vi "ALEX.vi"(1 "Frame Number\n(starts with 1)":i32, 2 "ALEX?":bool, 3 "Shutter Enable":bool[](array[boolean])) -> (0 "Shutter State":bool[](array[boolean]))   [LabVIEW 2023, in "NI DAQ.lvlib" / "NI DAQ.lvclass"]
uses:
  NI DAQ.lvclass
  NI DAQ.lvclass/NI DAQ.ctl
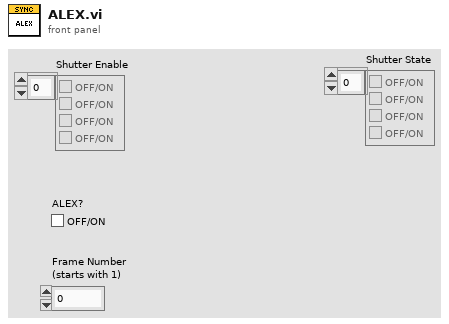
[diagram p1: front panel]
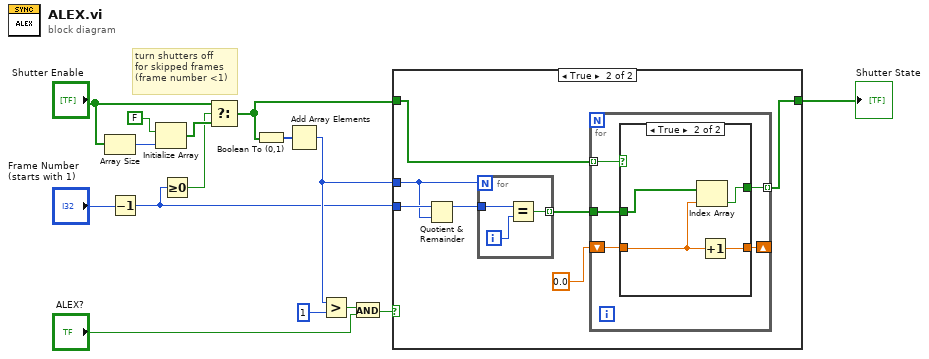
[diagram p0: block diagram]
diagram:
  # "turn shutters off\nfor skipped frames\n(frame number <1)"
  n1 = Array Size(array="Shutter Enable") -> (size(s)=w4:i32)
  n2 = Decrement(x="Frame Number\n(starts with 1)") -> (x-1=w2:i32)
  n3 = Initialize Array(FALSE, w4) -> (w6:bool[])
  n4 = Greater Or Equal To 0?(x=w2) -> (x >= 0?=w1:bool)
  n5 = Select(t="Shutter Enable", s=w1, f=w6) -> (s? t:f=w7:bool[])
  n6 = Boolean To (0,1)(Boolean=w7) -> (0, 1=w14:i16[])
  n7 = Add Array Elements(numeric array=w14) -> (sum=w11:i16)
  n8 = Greater?(x=w11, y=i16 1) -> (0:w12:bool)
  n9 = And(x=w12, y="ALEX?") -> (x .and. y?=w13:bool)
  n10 = case shown="True" w13 {
    tunnel: w7 -> [w16 w18]
    tunnel: w2 -> [_ w23]
    tunnel: [w16 w17] -> w15
    tunnel: w11 -> [_ w22]
    frame False {
    }
    frame True {
      n11 = Quotient & Remainder(x=w23, y=w22) -> (x-y*floor(x/y)=w21:i32)  [unwired: 1 out]
      n12 = for {
        N: w22 -> [_]
        tunnel: w21 -> [w37]
        tunnel: [w35] -> w19 mode=indexing
        i -> [w36]
        n13 = Equal?(x=w37, y=w36) -> (x = y?=w35:bool)
      }
      n14 = for {
        tunnel: w18 -> [w28] mode=indexing
        tunnel: w19 -> [w26]
        tunnel: [w27] -> w17 mode=indexing
        shift-right: [w24] -> _
        shift-left: 0.0 ("x") -> [w25]
        n15 = case shown="True" w28 {
          selector: w28 -> [w30 _]
          tunnel: [w30 w33] -> w27
          tunnel: w26 -> [_ w34]
          tunnel: w25 -> [w29 w31]
          tunnel: [w29 w32] -> w24
          frame False {
          }
          frame True {
            n16 = Index Array(array=w34, index=w31) -> (element=w33:bool)
            n17 = Increment(x=w31) -> (x+1=w32:dbl)
          }
        }
      }
    }
  }
  "Shutter State" <- w15
